vi "PH_gentec_Powermeter.PC Set Zero.vi"(0 "VI in":refnum<vi>, 2 "Set Zero":bool, 5 "error in (no error)":errorcluster) -> (14 "VI out":refnum<vi>, 19 "error out":errorcluster)   [LabVIEW 2014, in "PH_gentec_Powermeter.lvlib"]
uses:
  PH_gentec_Powermeter.lvlib
  PH_Basics/PH_Common/PH_Common.lvlib
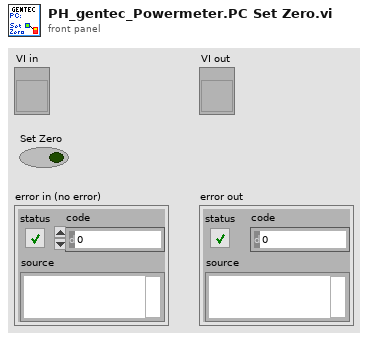
[diagram p1: front panel]
types:
  T1 = typedef "PH_gentec_Powermeter.lvlib/PH_gentec_Powermeter.i attribute.ctl" = cluster{"GUI References":cluster{"delete":refnum<vi>, "start stop Statistics":refnum<vi>, "Statistic Data":refnum<vi>, "Configuration Values":refnum<vi>, "Set Zero":refnum<vi>, "Data Sampling Settings":refnum<vi>, "Wanted Sets":refnum<vi>, "Current Sets":refnum<vi>}, "Start Stop Statistics":bool, "Wanted Sets":T2, "Current Sets":T2}
  T2 = typedef "PH_gentec_Powermeter.lvlib/PH_gentec_Powermeter.Sets.ctl" = cluster{"Data Sampling Settings":T3, "Set Zero":bool}
  T3 = typedef "gentec-SOLO-PE - Driver.lvlib/gentec-SOLO-PE.Data Sampling Settings.ctl" = cluster{"Sample Rate":u32, "Sample Rate Unit":u32, "Sample Period":u32, "Sample Period Unit":u32, "Total Duration":u32, "Total Duration Unit":u32, "Time Stamp":u32}
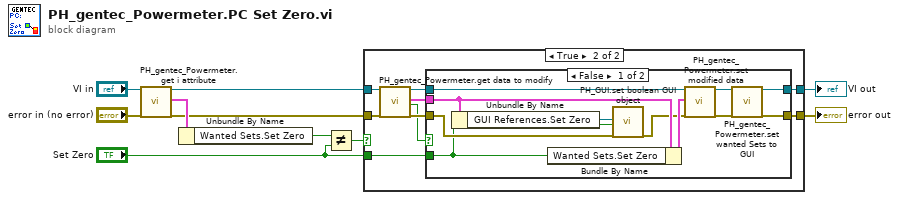
[diagram p0: block diagram]
diagram:
  n1 = call "PH_gentec_Powermeter.get i attribute.vi"("i ref in"="VI in", "error in (no error)"="error in (no error)") -> ("i ref out"=w6:refnum<vi>, "i attribute"=w7:T1, "error out"=w4:errorcluster)  [unwired: 15 in]
  n2 = Unbundle By Name(w7) -> ("Wanted Sets.Set Zero"=w8:bool)
  n3 = Not Equal?(x=w8, y="Set Zero") -> (x != y?=w10:bool)
  n4 = case shown="True" w10 {
    tunnel: [w11 w20] -> w2
    tunnel: [w12 w18] -> w3
    tunnel: w4 -> [w11 w15]
    tunnel: w6 -> [w12 w14]
    tunnel: "Set Zero" -> [_ w13]
    frame False {
    }
    frame True {
      n5 = call "PH_gentec_Powermeter.get data to modify.vi"("i ref in"=w14, "error in (no error)"=w15) -> ("i ref out"=w19:refnum<vi>, "i attribute"=w17:T1, "timed out"=w16:bool, "error out"=w21:errorcluster)  [unwired: 14 in]
      n6 = case shown="False" w16 {
        tunnel: w21 -> [w32 w33]
        tunnel: [w24 w33] -> w20
        tunnel: w19 -> [w31 w34]
        tunnel: [w22 w34] -> w18
        tunnel: w17 -> [w29 _]
        tunnel: w13 -> [w26 _]
        frame False {
          n7 = Unbundle By Name(w29) -> ("GUI References.Set Zero"=w27:refnum<vi>)
          n8 = Bundle By Name(cluster=w29, "Wanted Sets.Set Zero"=w26) -> (w30:T1)
          n9 = call "PH_GUI.set boolean GUI object.vi"("Boolean Knob GUI Ref"=w27, "Value"=w26, "error in (no error)"=w32) -> ("error out"=w28:errorcluster)  [unwired: 16 in]
          n10 = call "PH_gentec_Powermeter.set modified data.vi"("i ref in"=w31, "i attribute"=w30, "error in (no error)"=w28) -> ("i ref out"=w23:refnum<vi>, "error out"=w25:errorcluster)  [unwired: 15 in]
          n11 = call "PH_gentec_Powermeter.set wanted Sets to GUI.vi"("i ref in"=w23, "error in"=w25) -> ("i ref out"=w22:refnum<vi>, "error out"=w24:errorcluster)  [unwired: 16 in]
        }
        frame True {
        }
      }
    }
  }
  "VI out" <- w3
  "error out" <- w2
